vi "DrivetrainControl.vi"(11 "HMI to Control":T1={"RightDriveValue"=0.0, "LeftDriveValue"=0.0, "Arm Manual "=0.0, "Stacker Manual "=0.0, "Claw Manual "=0.0, "ClawSlightOpenNumber"=0, "Intake Value "=0.0, "Arm States"=enum."4 Tote", "Claw States"=enum."Claw Manual ", "Intake Man. or Sense"=enum."Sensing", "Stacker in Manual?"=FALSE, "Drop Stack? "=FALSE, "Tusk Up Request"=FALSE, "Tusk Down Request"=FALSE, "Inver. Wheels  In Request"=FALSE, "Inverse. Wheels Out Request "=FALSE, "Get Out of Manual Control"=FALSE, "Exit Score State"=FALSE, "DriveStraight Help?"=FALSE, "Stacker Shut Off No."=0, "Stacker Need Off?"=FALSE, "Collecting?"=FALSE, "Go to Hover"=FALSE, "Stack Clamp Lock "=FALSE, "Stack Clamp Unlock "=FALSE, "Claw Intake Value "=0.0, "Stack Clamp Lock No. "=0, "Steal Can (ruin their day?)"=FALSE, "Retract (have mercy?)"=FALSE, "Can Grab No. "=0, "Wench Value to Control "=0.0}) -> (2 "LeftDriveFinalOutput":dbl format="%#_13g", 3 "RightDriveFinalOutput":dbl format="%#_13g")   [LabVIEW 2014]
uses:
  Typedefs/HMI_to_Control.ctl
  Typedefs/Arm States.ctl
  Typedefs/ClawStates.ctl
  Typedefs/IntakeWheelSenseOrManual.ctl
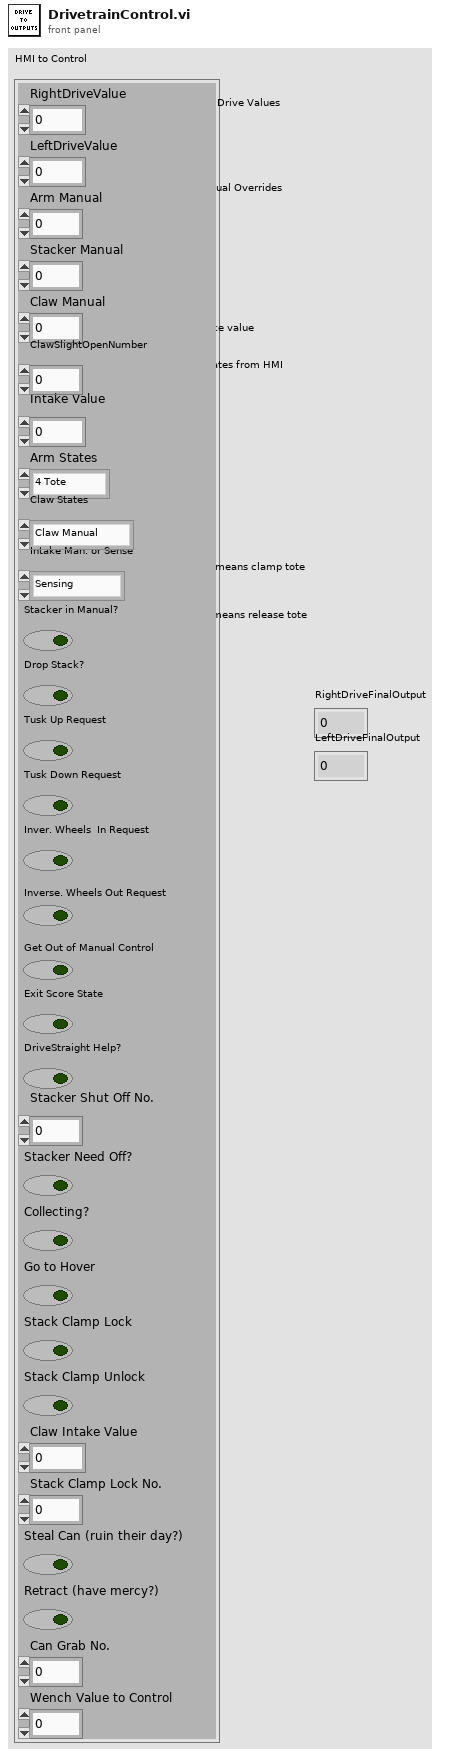
[diagram p1: front panel]
types:
  T1 = typedef "HMI_to_Control.ctl" = cluster{"RightDriveValue":dbl, "LeftDriveValue":dbl, "Arm Manual ":dbl, "Stacker Manual ":dbl, "Claw Manual ":dbl, "ClawSlightOpenNumber":i8, "Intake Value ":sgl, "Arm States":T2, "Claw States":T3, "Intake Man. or Sense":T4, "Stacker in Manual?":bool, "Drop Stack? ":bool, "Tusk Up Request":bool, "Tusk Down Request":bool, "Inver. Wheels  In Request":bool, "Inverse. Wheels Out Request ":bool, "Get Out of Manual Control":bool, "Exit Score State":bool, "DriveStraight Help?":bool, "Stacker Shut Off No.":i8, "Stacker Need Off?":bool, "Collecting?":bool, "Go to Hover":bool, "Stack Clamp Lock ":bool, "Stack Clamp Unlock ":bool, "Claw Intake Value ":sgl, "Stack Clamp Lock No. ":i8, "Steal Can (ruin their day?)":bool, "Retract (have mercy?)":bool, "Can Grab No. ":i8, "Wench Value to Control ":dbl}
  T2 = typedef "Arm States.ctl" = enum16{"Arm Manual ", "Ground", "Step", "1 Tote", "2 Tote", "3 Tote", "4 Tote", "5 Tote", "6 Tote", "Flip Can Arm", "Grab Can in auto", "Nudge"}
  T3 = typedef "ClawStates.ctl" = enum16{"Claw Manual ", "Claw Open", "Claw Closed", "Claw Slight Open", "Flip Can"}
  T4 = typedef "IntakeWheelSenseOrManual.ctl" = enum16{"Sensing", "Manual "}
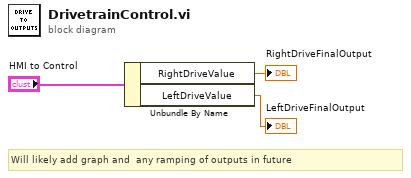
[diagram p0: block diagram]
diagram:
  # "Will likely add graph and  any ramping of outputs in future"
  n1 = Unbundle By Name("HMI to Control") -> ("RightDriveValue"=→"RightDriveFinalOutput":dbl, "LeftDriveValue"=→"LeftDriveFinalOutput":dbl)
